vi "MGI Wrap String to Pixel Width.vi"(1 "Width":i16, 2 "String":string, 3 "Font":T1) -> (0 "Wrapped String":string)   [LabVIEW 2020]
doc: "Add line feeds to the specified string to wrap it to the specified width.\n\nAuthored by David A. Moore\nsupport@mooregoodideas.com\nwww.mooregoodideas.com\n\nCopyright (c) 2010, Moore Good Ideas, Inc.\n\nAll rights reserved.\n\nRedistribution and use in source and binary forms, with or without modification, are permitted provided that the following conditions are met:\n\n * Redistributions of source code must retain the above copyright notice, this list of conditions and the following disclaimer.\n * Redistributions in binary form must reproduce the above copyright notice, this list of conditions and the following disclaimer in the documentation and/or other materials provided with the distribution.\n * Neither the name of Moore Good Ideas, Inc. nor the names of its contributors may be used to endorse or promote products derived from this software without specific prior written permission.\n\nTHIS SOFTWARE IS PROVIDED BY THE COPYRIGHT HOLDERS AND CONTRIBUTORS \"AS IS\" AND ANY EXPRESS OR IMPLIED WARRANTIES, INCLUDING, BUT NOT LIMITED TO, THE IMPLIED WARRANTIES OF MERCHANTABILITY AND FITNESS FOR A PARTICULAR PURPOSE ARE DISCLAIMED. IN NO EVENT SHALL THE COPYRIGHT OWNER OR CONTRIBUTORS BE LIABLE FOR ANY DIRECT, INDIRECT, INCIDENTAL, SPECIAL, EXEMPLARY, OR CONSEQUENTIAL DAMAGES (INCLUDING, BUT NOT LIMITED TO, PROCUREMENT OF SUBSTITUTE GOODS OR SERVICES; LOSS OF USE, DATA, OR PROFITS; OR BUSINESS INTERRUPTION) HOWEVER CAUSED AND ON ANY THEORY OF LIABILITY, WHETHER IN CONTRACT, STRICT LIABILITY, OR TORT (INCLUDING NEGLIGENCE OR OTHERWISE) ARISING IN ANY WAY OUT OF THE USE OF THIS SOFTWARE, EVEN IF ADVISED OF THE POSSIBILITY OF SUCH DAMAGE."
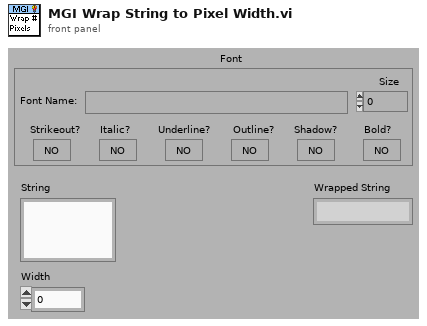
[diagram p1: front panel]
types:
  T1 = cluster{"Font Name:":string, "Size":i16, "Strikeout?":bool, "Italic?":bool, "Underline?":bool, "Outline?":bool, "Shadow?":bool, "Bold?":bool}
  T2 = enum16{"User-specified Font", "Application Font", "System Font", "Dialog Font"}
  T3 = cluster{"left":i16, "top":i16, "right":i16, "bottom":i16}
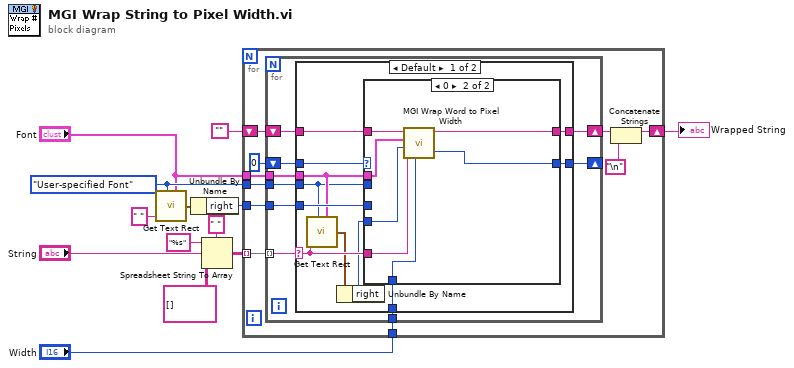
[diagram p0: block diagram]
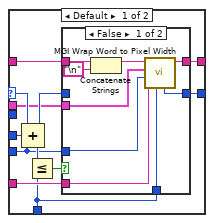
[diagram p2: hidden frame]
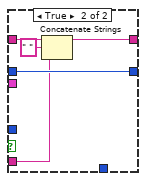
[diagram p3: hidden frame]
diagram:
  w4 = T2."User-specified Font" ("desired font(application)")
  n1 = call <vilib>:"Get Text Rect.vi"("desired font(Application)"=w4, "text"=" ", "[user-specified font]"="Font") -> ("rect"=w6:T3)  [unwired: 6 in]
  n2 = Unbundle By Name(w6) -> ("right"=w5:i16)
  n3 = Spreadsheet String To Array(delimiter (Tab)=" ", format string="%s", spreadsheet string="String", array type (2D Dbl)=string[][] []) -> (array=w9:string[][])
  n4 = for {
    tunnel: w9 -> [w23] mode=indexing
    shift-right: [w18] -> w2
    shift-left: "" -> [w22]
    tunnel: w5 -> [w15]
    tunnel: w4 -> [w17]
    tunnel: "Font" -> [w16]
    tunnel: "Width" -> [w14]
    n5 = for {
      tunnel: w23 -> [w32] mode=indexing
      shift-right: [w30] -> w20
      shift-left: w22 -> [w31]
      shift-right: [w28] -> _
      shift-left: i16 0 ("right") -> [w29]
      tunnel: w17 -> [w27]
      tunnel: w16 -> [w26]
      tunnel: w15 -> [w25]
      tunnel: w14 -> [w24]
      n6 = case shown="Default" w32 {
        selector: w32 -> [w40 _]
        tunnel: w31 -> [w42 w77]
        tunnel: [w41 w77] -> w30
        tunnel: w29 -> [w43 w76]
        tunnel: [w36 w76] -> w28
        tunnel: w27 -> [w33 _]
        tunnel: w26 -> [w34 _]
        tunnel: w25 -> [w39 _]
        tunnel: w24 -> [w35 _]
        frame Default {
          n7 = call <vilib>:"Get Text Rect.vi"("desired font(Application)"=w33, "text"=w40, "[user-specified font]"=w34) -> ("rect"=w38:T3)  [unwired: 6 in]
          n8 = Unbundle By Name(w38) -> ("right"=w37:i16)
          n9 = case shown="0" w43 {
            selector: w43 -> [w54 _]
            tunnel: w42 -> [w49 w75]
            tunnel: [w46 w74] -> w41
            tunnel: w40 -> [w50 w71]
            tunnel: w39 -> [w53 _]
            tunnel: w37 -> [w48 w70]
            tunnel: [w47 w69] -> w36
            tunnel: w35 -> [w44 w72]
            tunnel: w34 -> [w45 w73]
            tunnel: w33 -> [_ _]
            frame Default {
              n10 = Compound Arithmetic op=ADD(w54, w53, w48) -> (w52:i16)
              n11 = Less Or Equal?(x=w52, y=w44) -> (x <= y?=w51:bool)
              n12 = case shown="False" w51 {
                tunnel: w50 -> [w60 w65]
                tunnel: w49 -> [w63 w67]
                tunnel: w48 -> [w59 _]
                tunnel: w52 -> [_ w68]
                tunnel: [w55 w68] -> w47
                tunnel: [w56 w66] -> w46
                tunnel: w45 -> [w58 _]
                tunnel: w44 -> [w57 _]
                frame False {
                  n13 = Concatenate Strings(w63, "\n") -> (w61:string)
                  n14 = call <userlib>:"MGI Wrap Word to Pixel Width.vi"("Allowed Width"=w57, "Word"=w60, "Word Width(pixels)"=w59, "Font"=w58, "Start String"=w61) -> ("String Out"=w56:string, "Width Used"=w55:i16)  [unwired: 5 in]
                }
                frame True {
                  n15 = Concatenate Strings(w67, " " ("Substring"), w65) -> (w66:string)
                }
              }
            }
            frame 0 {
              n16 = call <userlib>:"MGI Wrap Word to Pixel Width.vi"("Allowed Width"=w72, "Word"=w71, "Word Width(pixels)"=w70, "Font"=w73, "Start String"=w75) -> ("String Out"=w74:string, "Width Used"=w69:i16)  [unwired: 5 in]
            }
          }
        }
        frame "" {
        }
      }
    }
    n17 = Concatenate Strings(w20, "\n") -> (w18:string)
  }
  "Wrapped String" <- w2
